vi "Get Base Path.vi"(6 "Strip lead \"/\" (F)":bool, 8 "error in (no error)":errorcluster, 11 "URI in":refnum<class "URI.lvclass">) -> (0 "error out":errorcluster, 2 "base-path":string, 3 "URI out":refnum<class "URI.lvclass">)   [LabVIEW 2013, in "openURI.lvlib" / "URI.lvclass"]
uses:
  URI.lvclass
  URI.lvclass/URI.ctl
  components/path/URI-Component.Path.lvclass
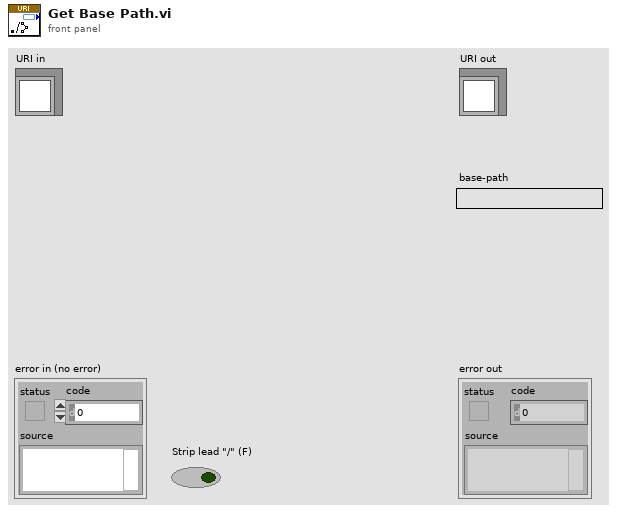
[diagram p1: front panel]
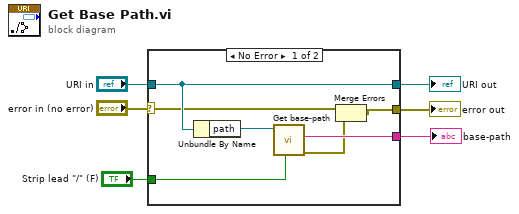
[diagram p0: block diagram]
diagram:
  n1 = case shown="No Error" "error in (no error)" {
    selector: "error in (no error)" -> [w12 w15]
    tunnel: [w11 w15] -> w5
    tunnel: [w13 w14] -> w3
    tunnel: "URI in" -> [w13 w14]
    tunnel: [w8 _] -> w2
    tunnel: "Strip lead \"/\" (F)" -> [w9 _]
    frame No Error {
      n2 = Unbundle By Name(w13) -> ("path"=w10:refnum<class "URI-Component.Path.lvclass">)
      n3 = call "Get base-path.vi"("Strip lead \"/\" (F)"=w9, "URI-Component.Path in"=w10) -> ("error out"=w7:errorcluster, "base-path"=w8:string)  [unwired: 7 in, 1 out]
      n4 = Merge Errors(w12, w7) -> (w11:errorcluster)
    }
    frame Error {
    }
  }
  "error out" <- w5
  "URI out" <- w3
  "base-path" <- w2
